vi "TopLevel.vi"() -> ()   [LabVIEW 2020]
uses:
  Project/DowntimeReport/StateMachineTypedef.ctl
  <vilib>/Utility/miscctls.llb/LVRowAndColumnTypeDef.ctl
  d59d2eb3-6a34-4e13-8a79-7d27c84295cb.vi
  <vilib>/Utility/file.llb/Read Delimited Spreadsheet (string).vi
panel:
  out "Events":i32
  in  "Load":bool
  out "Table Out":string[][](table)
  in  "Listbox":i32(listbox)
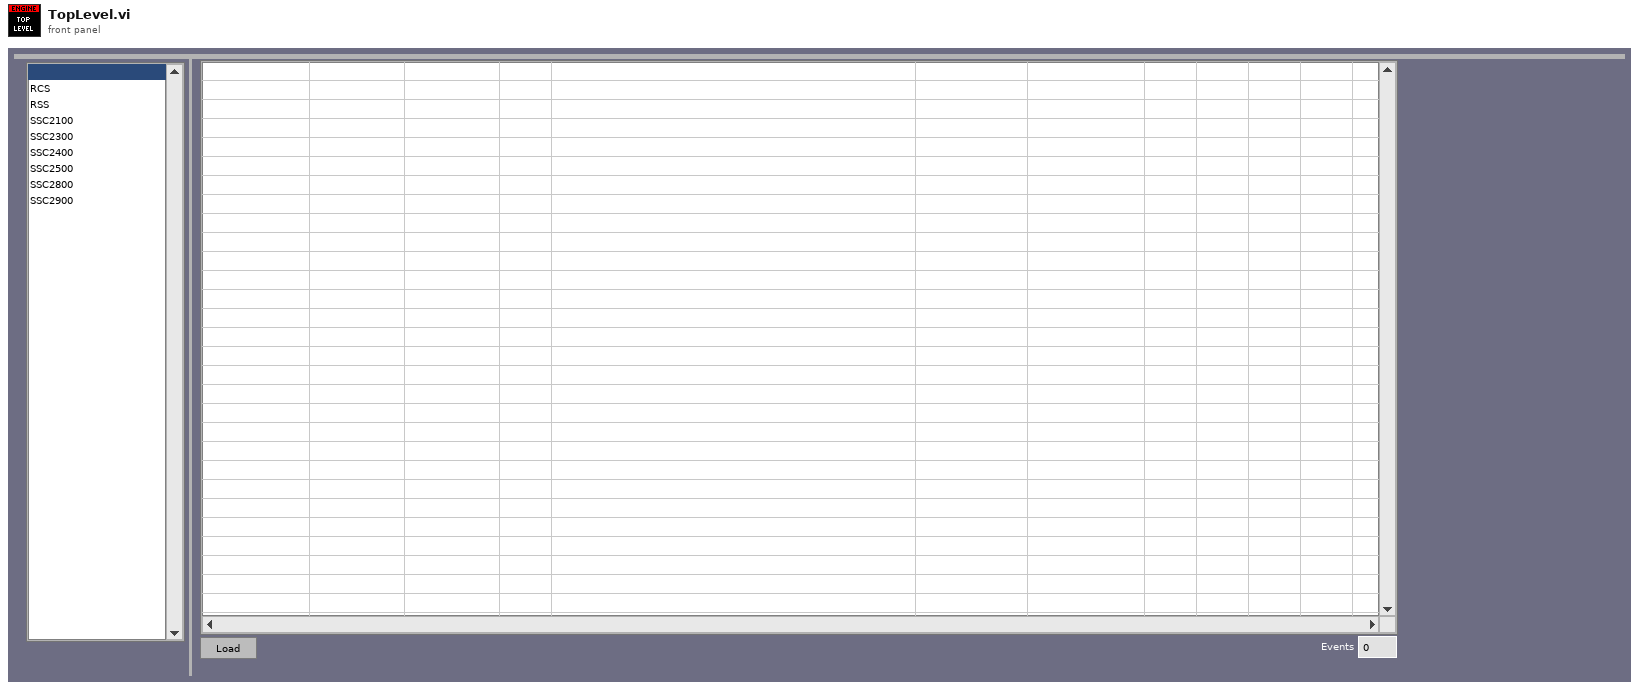
[diagram p1: front panel]
types:
  T1 = cluster{"Sheets":string[][][], "SSC Names":string[], "Selected":i32}
  T2 = typedef "StateMachineTypedef.ctl" = enum16{"Init", "Wait", "UpdateIndicators", "UpdateControls", "Terminate"}
  T3 = typedef "LVRowAndColumnTypeDef.ctl" = cluster{"Row":i32, "Column":i32}
  T4 = enum8{"Enabled", "Disabled", "Disabled and Grayed Out"}
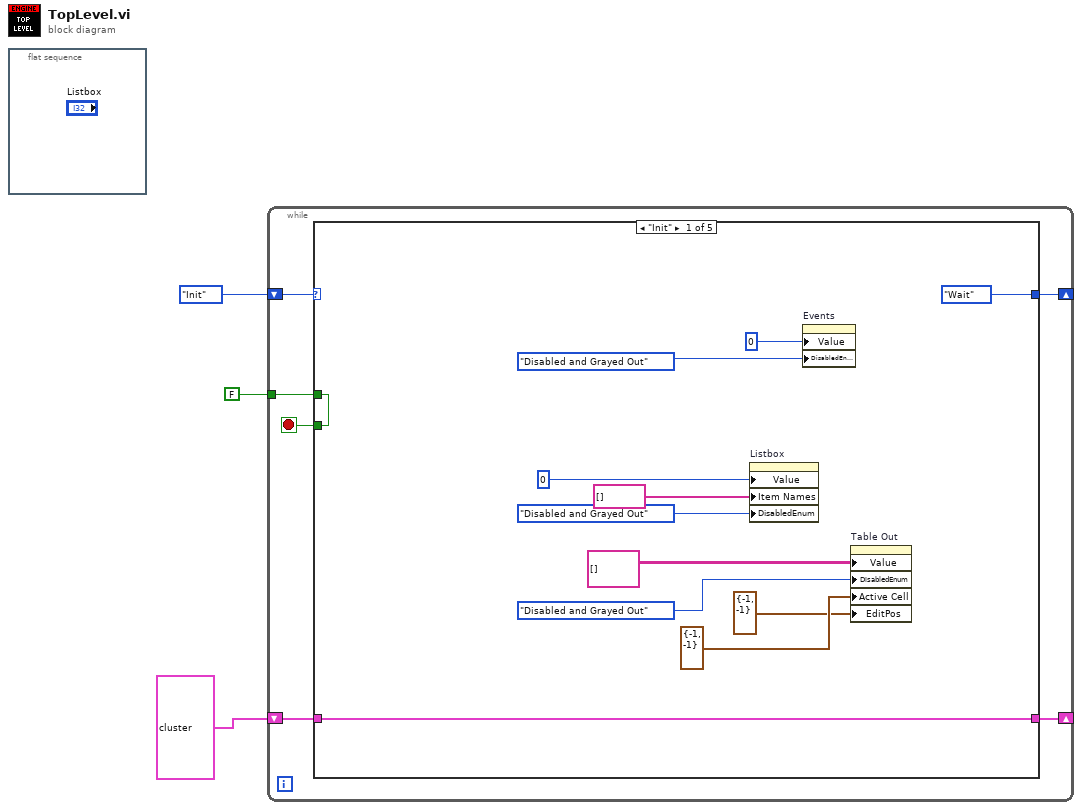
[diagram p0: block diagram]
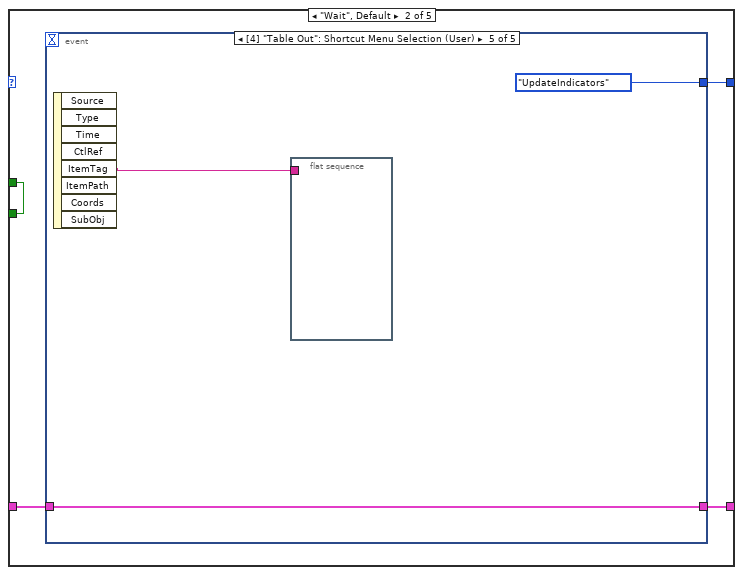
[diagram p2: hidden frame]
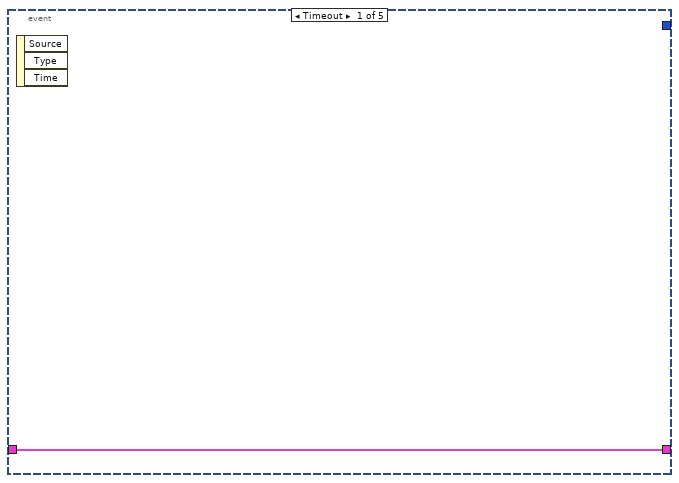
[diagram p3: hidden frame]
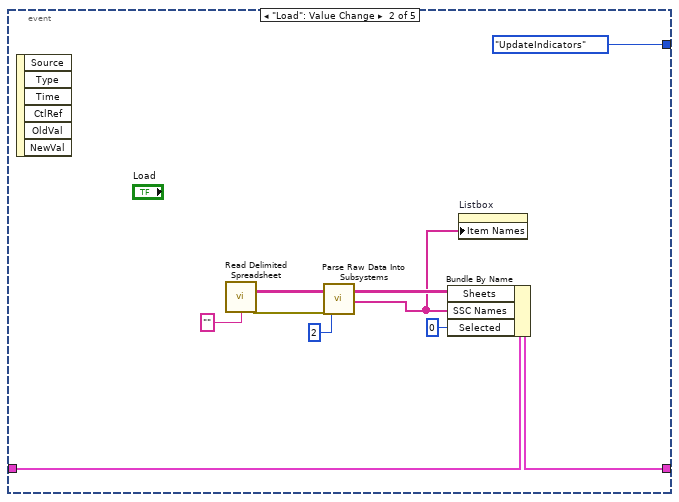
[diagram p4: hidden frame]
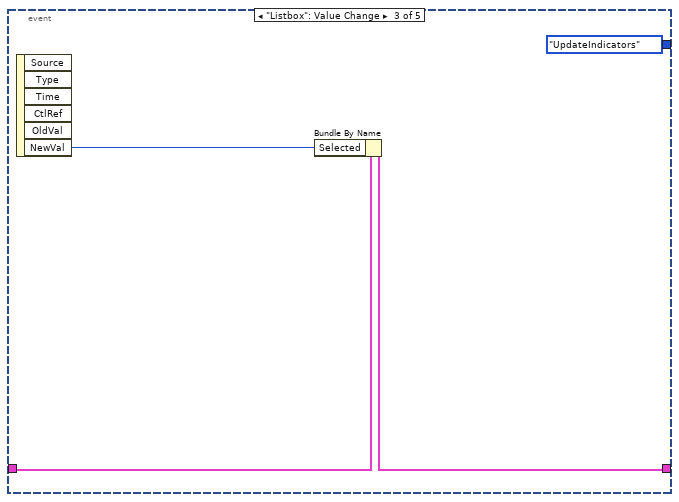
[diagram p5: hidden frame]
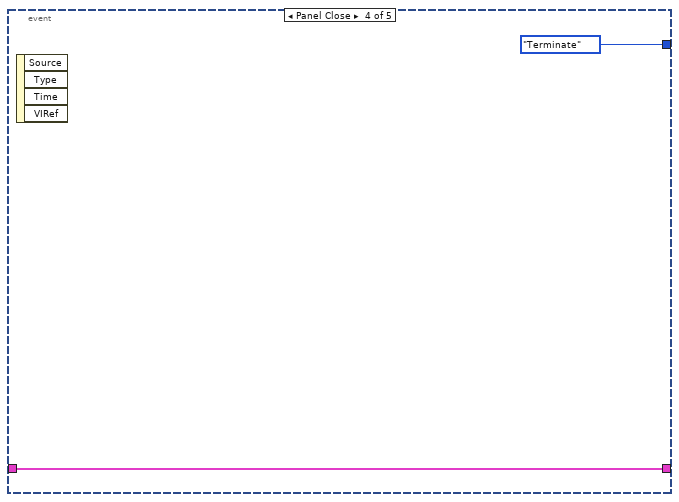
[diagram p6: hidden frame]
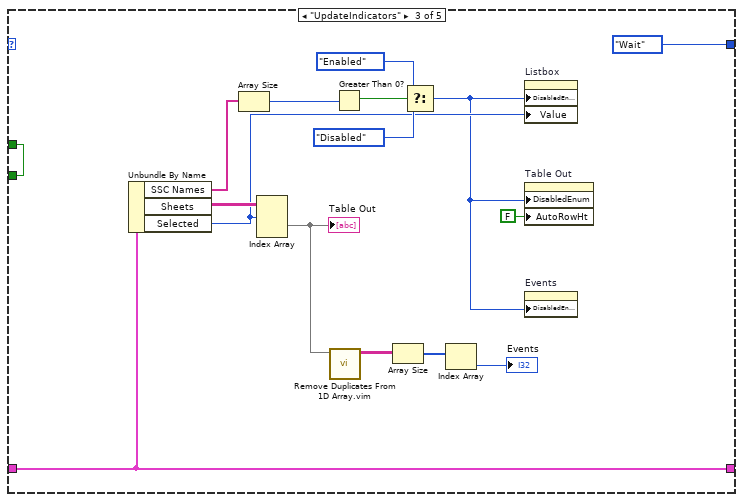
[diagram p7: hidden frame]
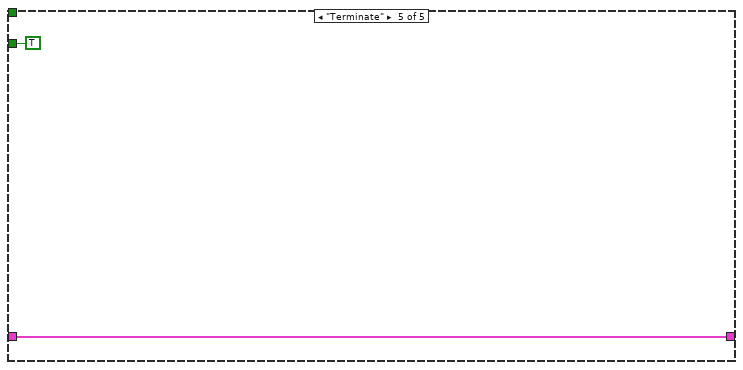
[diagram p9: hidden frame]
diagram:
  n1 = flat-sequence {
    frame #0 {
    }
  }
  n2 = while {
    shift-right: [w8] -> _
    shift-left: StateMachineTypedef."Init" -> [w9]
    shift-right: [w6] -> _
    shift-left: T1 {"Sheets"=array10x19805x10[1980500 elements], "SSC Names"=[], "Selected"=0} -> [w7]
    tunnel: FALSE -> [w5]
    stop <- w4 stop-if-true
    n3 = case shown="\"Init\"" w9 {
      tunnel: [StateMachineTypedef."Wait" w25 StateMachineTypedef."Wait" _ _] -> w8
      tunnel: w7 -> [w16 w24 w60 w63 w65]
      tunnel: [w16 w23 w60 w63 w65] -> w6
      tunnel: w5 -> [w15 w22 w61 w62 _]
      tunnel: [w15 w22 w61 w62 TRUE] -> w4
      frame "Init" {
        n4 = property on="Listbox" class="LstBox (strict)"("Value"=0 ("Listbox"), "Item Names"=string[] [], "DisabledEnum"=T4."Disabled and Grayed Out" ("Disabled")) -> ()  [unwired: 2 in, 2 out]
        n5 = property on="Events" class="DigNum (strict)"("Value"=0 ("Events"), "DisabledEnum"=T4."Disabled and Grayed Out" ("Disabled")) -> ()  [unwired: 2 in, 2 out]
        n6 = property on="Table Out" class="Tbl (strict)"("Value"=string[][] [] ("Table Out"), "DisabledEnum"=T4."Disabled and Grayed Out" ("Disabled"), "Active Cell"=T3 {"Row"=-1, "Column"=-1} ("Active Cell:Active Cell"), "EditPos"=T3 {"Row"=-1, "Column"=-1} ("Edit Position")) -> ()  [unwired: 2 in, 2 out]
      }
      frame "Wait", Default {
        n7 = event shown="[4] \"Table Out\": Shortcut Menu Selection (User)" {
          selector: _ -> [_ _ _ _ _]
          dyn-events: _ -> [_ _ _ _ _]
          timeout: _ -> [_ _ _ _ _]
          tunnel: [_ StateMachineTypedef."UpdateIndicators" StateMachineTypedef."UpdateIndicators" StateMachineTypedef."Terminate" StateMachineTypedef."UpdateIndicators"] -> w25
          tunnel: w24 -> [w26 w33 w39 w42 w44]
          tunnel: [w26 w32 w38 w42 w44] -> w23
          event Timeout {
            n8 = event-data() -> ()  [unwired: 1 in, 3 out]
          }
          event "Load": Value Change {
            n9 = event-data() -> ()  [unwired: 1 in, 6 out]
            n10 = call-poly <vilib>:"Read Delimited Spreadsheet.vi"("delimiter (\\t)"="" ("delimiter (\\t)")) -> ("all rows"=w35:string[][], "error out"=w34:errorcluster)  [unwired: 9 in, 4 out]
            n11 = call "Parse Raw Data Into Subsystems.vi"("Table In"=w35, "Error In"=w34, "SSC Column"=2) -> ("Tables Out"=w31:string[][][], "SSC Names"=w29:string[])  [unwired: 14 in, 1 out]
            n12 = Bundle By Name(cluster=w33, "Sheets"=w31, "SSC Names"=w29, "Selected"=0) -> (w32:T1)
            n13 = property on="Listbox" class="LstBox (strict)"("Item Names"=w29) -> ()  [unwired: 2 in, 2 out]
          }
          event "Listbox": Value Change {
            n14 = event-data() -> ("NewVal"=w37:i32)  [unwired: 1 in, 5 out]
            n15 = Bundle By Name(cluster=w39, "Selected"=w37) -> (w38:T1)
          }
          event Panel Close {
            n16 = event-data() -> ()  [unwired: 1 in, 4 out]
          }
          event "Table Out": Shortcut Menu Selection (User) {
            n17 = event-data() -> ("ItemTag"=w43:string)  [unwired: 1 in, 7 out]
            n18 = flat-sequence {
              tunnel: w43 -> [_]
              frame #0 {
              }
            }
          }
        }
      }
      frame "UpdateIndicators" {
        n19 = Unbundle By Name(w60) -> ("SSC Names"=w57:string[], "Sheets"=w59:string[][][], "Selected"=w52:i32)
        n20 = Array Size(array=w57) -> (size(s)=w58:i32)
        n21 = Index Array(array=w59, index (dim 0)=w52) -> (element=w48:string[][])  [unwired: 2 in]
        "Table Out" <- w48
        n22 = call "Remove Duplicates From 1D Array.vim"("array"=w48) -> ("array with duplicates removed"=w47:string[][])  [unwired: 10 in]
        n23 = Greater Than 0?(x=w58) -> (x > 0?=w56:bool)
        n24 = Array Size(array=w47) -> (size(s)=w50:i32[])
        n25 = Select(t=T4."Enabled" ("Disabled"), s=w56, f=T4."Disabled" ("Disabled")) -> (s? t:f=w46:T4)
        n26 = Index Array(array=w50) -> (element=→"Events":i32)  [unwired: 1 in]
        n27 = property on="Listbox" class="LstBox (strict)"("DisabledEnum"=w46, "Value"=w52) -> ()  [unwired: 2 in, 2 out]
        n28 = property on="Table Out" class="Tbl (strict)"("DisabledEnum"=w46, "AutoRowHt"=FALSE ("Autosizing Row Height")) -> ()  [unwired: 2 in, 2 out]
        n29 = property on="Events" class="DigNum (strict)"("DisabledEnum"=w46) -> ()  [unwired: 2 in, 2 out]
      }
      frame "UpdateControls" {
      }
      frame "Terminate" {
      }
    }
  }
